vi "MeasureAtFreq.vi"(8 "error in (no error)":errorcluster, 10 "Frequency (Hz)":dbl, 11 "PwrMtr_RSNRPZ in":refnum<class "PwrMtr_RSNRPZ.lvclass">) -> (0 "error out":errorcluster, 2 "Power (dBm)":dbl, 3 "PwrMtr_RSNRPZ out":refnum<class "PwrMtr_RSNRPZ.lvclass">)   [LabVIEW 2014, in "PwrMtr_RSNRPZ.lvclass"]
uses:
  PwrMtr_RSNRPZ.lvclass
  PwrMtr_RSNRPZ.lvclass/PwrMtr_RSNRPZ.ctl
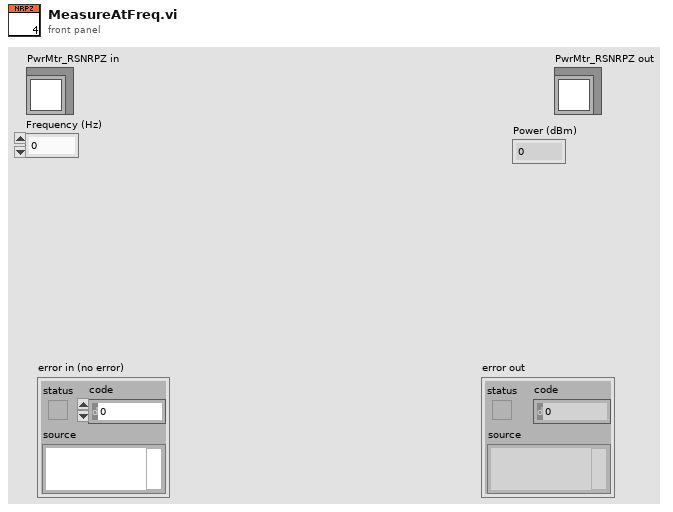
[diagram p1: front panel]
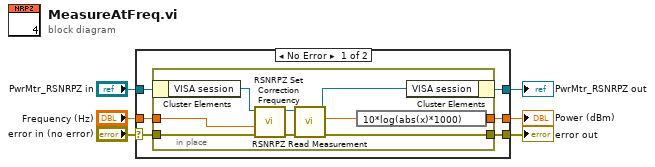
[diagram p0: block diagram]
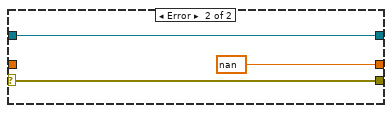
[diagram p2: hidden frame]
diagram:
  n1 = case shown="No Error" "error in (no error)" {
    selector: "error in (no error)" -> [w12 w23]
    tunnel: "Frequency (Hz)" -> [w10 _]
    tunnel: "PwrMtr_RSNRPZ in" -> [w8 w24]
    tunnel: [w11 w23] -> w4
    tunnel: [w9 nan ("Amplitude (Cal)")] -> w3
    tunnel: [w7 w24] -> w1
    frame No Error {
      n2 = in-place {
        in-place-border: w12 -> [w21]
        in-place-border: [w20] -> w11
        in-place-border: w10 -> [w19]
        in-place-border: [w13] -> w9
        n3 = in-place-cluster #1(w8) -> ("VISA session"=w18:refnum<visa-resource-name>)
        n4 = call "RSNRPZ Set Correction Frequency.vi"("error in (no error)"=w21, "Frequency ( 50.0e6 Hz)"=w19, "VISA session"=w18) -> ("error out"=w16:errorcluster, "dup VISA session"=w15:refnum<visa-resource-name>)  [unwired: 7 in]
        n5 = call "RSNRPZ Read Measurement.vi"("error in (no error)"=w16, "VISA session"=w15) -> ("error out"=w20:errorcluster, "Measurement"=w14:dbl, "dup VISA session"=w17:refnum<visa-resource-name>)  [unwired: 7 in]
        n6 = expression code="10*log(abs(x)*1000)"(w14) -> (w13:dbl)
        n7 = in-place-cluster #1("VISA session"=w17) -> (w7:refnum<class "PwrMtr_RSNRPZ.lvclass">)
      }
    }
    frame Error {
    }
  }
  "error out" <- w4
  "Power (dBm)" <- w3
  "PwrMtr_RSNRPZ out" <- w1
